vi "CRYGet Information for ActiveX.vi"() -> (2 "Limit Array Out":string, 3 "Sequence Array Out":string)   [LabVIEW 2013]
uses:
  CRYProject/CRYProject Editor Global.vi
panel:
  out "Array":string[](array[string])
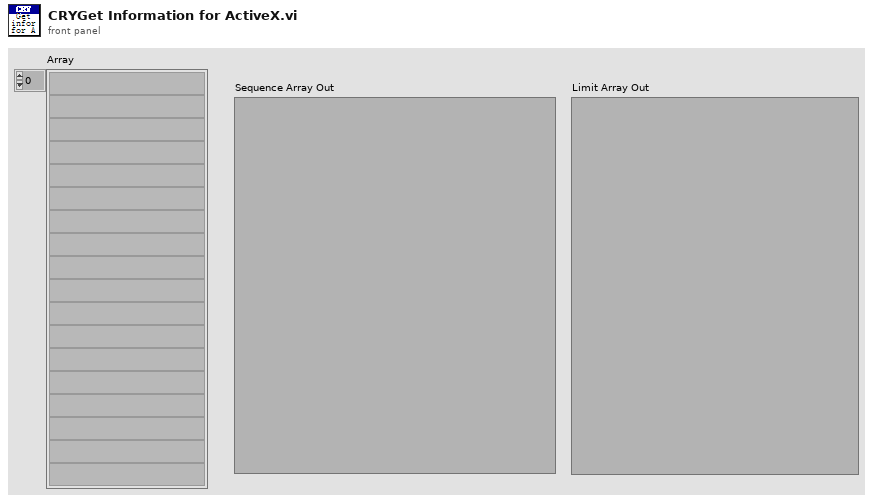
[diagram p1: front panel]
types:
  T1 = typedef "CRYStep.ctl" = cluster{"No.VI":i32, "Category":string, "StepName":string, "Seq setup flattened":string, "Comment":string, "Steps config.":bool[], "Jump config":i32[], "Start":dbl, "Increment":dbl, "Name":string, "Unit":string, "Y data":u16, "Y prefix":string, "Y dB ref":dbl, "Y unit":string, "Repeat State Array":cluster{"Start":dbl, "Increment":dbl, "Count":i32, "Num":i32}[]}
  T2 = typedef "CRYTS.ctl" = cluster{"No.TS":u16, "TS File Path":path, "TS Name":string, "EditStepName":string, "Steps":T1[], "New State":bool, "Change State":bool, "Flattened CurveLib Data":string, "Document Data":string, "EditStepNo":u16, "Operator Start File":string, "Sequence Type":string, "Sequence Language":string}
  T3 = typedef "CRYStimulus Cluster.ctl" = cluster{"StimulusType":string, "UseMLValArray":u16[], "ML_axisArray":u16[], "MLValLevelNameArray":string[], "Level(U)Array":dbl[], "Start(Stop)FreqArray":dbl[], "Start(Stop)AmpArray":dbl[], "StepResolutionArray":u16[], "Unit_Array":u16[], "DegValArray":dbl[], "DegUnitArray":string[], "Steps1":i32, "Cycle/step1(#)":u32, "Time/step1(s)":dbl, "Transition1":dbl, "SweepRate2":dbl, "Freq3(Hz)":dbl, "Steps3(#)":dbl, "Cycles3(#)":u32, "StepSize3":dbl, "wave time":string, "RMS_Value4":dbl, "Peak_Value4":dbl, "WavePath4":string, "RMS_unit4":string, "Peak_unit4":string, "wave Info":string, "dc_ctrl5_1":u16, "dc_ctrl5_2":u16, "dc_polar5":u16, "Max.Current":u16, "Steps5(#)":u32, "Time/Step5":dbl, "Level5":dbl, "StepsSize5Val":dbl, "StepSize5Unit":string, "SweepType":u16, "Fixed/Ratio6":u16, "Transition6":dbl, "Steps6(#)":dbl, "Cycle/Steps6(#)":u32, "Time/Steps6(s)":dbl, "Freq6(Hz)":dbl, "Difference6(Hz)":dbl, "Ratio6":string, "NoiseType7":u16, "Duration7(s)":dbl, "MinFreq7(Hz)":dbl, "MaxFreq7(Hz)":dbl, "MinFreq8(Hz)":dbl, "MaxFreq8(Hz)":dbl, "FreqRounding8":bool, "Duration8(s)":dbl, "Tones8":dbl, "RoundingVal8":dbl, "ApplyEQ":bool, "Duration(s)":dbl, "CustomStimulusName ":string, "Flatten Element Array":string[], "sine waves":cluster{"freq":dbl, "ampl":dbl, "cycles":dbl}[], "Channel Out":i32, "RatioVal6":dbl, "TabCtrl6":enum32{"Master Tone", "Slave Tone"}, "Signal Type Name":string, "Help":string, "Channel Sel":u16, "V on DUT":bool, "Output Imp":dbl, "Nominal Imp":dbl}
  T4 = typedef "CRYHardware Channel Info.ctl" = cluster{"ID":i32, "Name":string, "Digital":bool, "Input":bool, "Device Name":string, "Hardware Ch ID":u8, "Vmax (V)":dbl, "Latency (samples)":dbl, "Sampling Rate (Hz)":u32, "Bit Depth":u32, "Anti-aliasing Factor (%fs)":sgl, "DAQmx Channel":tag, "term config":i32, "Coupling":i32, "IEPE en":bool, "ASIOChannel Name":string, "Audio Driver":u16, "ASIOChannel Index":u8}
  T5 = typedef "CRYAcquisition Cluster.ctl" = cluster{"Mode":u16, "Name":string, "use ch name":bool, "Record Time":dbl, "hide rec":bool, "hide play":bool, "rec delay":dbl, "rec pad":dbl, "dcc units":i8, "sine gen setting":string, "scope_fft setting":string, "voltmeter setting":string, "rta setting":string, "trig offset(sec)":dbl, "triggered  record":bool, "trig level":dbl, "trig unit":u8, "trig slop":bool, "trig timeout(sec)":dbl, "add record":bool, "EQ":bool, "record table":string[][], "play table":string[][], "trig channel":string, "Help":string}
  T6 = typedef "CRYResult Cluster Array.ctl" = T7[]
  T7 = typedef "CRYResult Cluster.ctl" = cluster{"Name":string, "Margin":dbl, "unit":string, "Verdict":bool, "Limit":string, "Max/Min":string, "protected":bool, "Step No.":i32, "Test Info":string, "AutoProtect":bool}
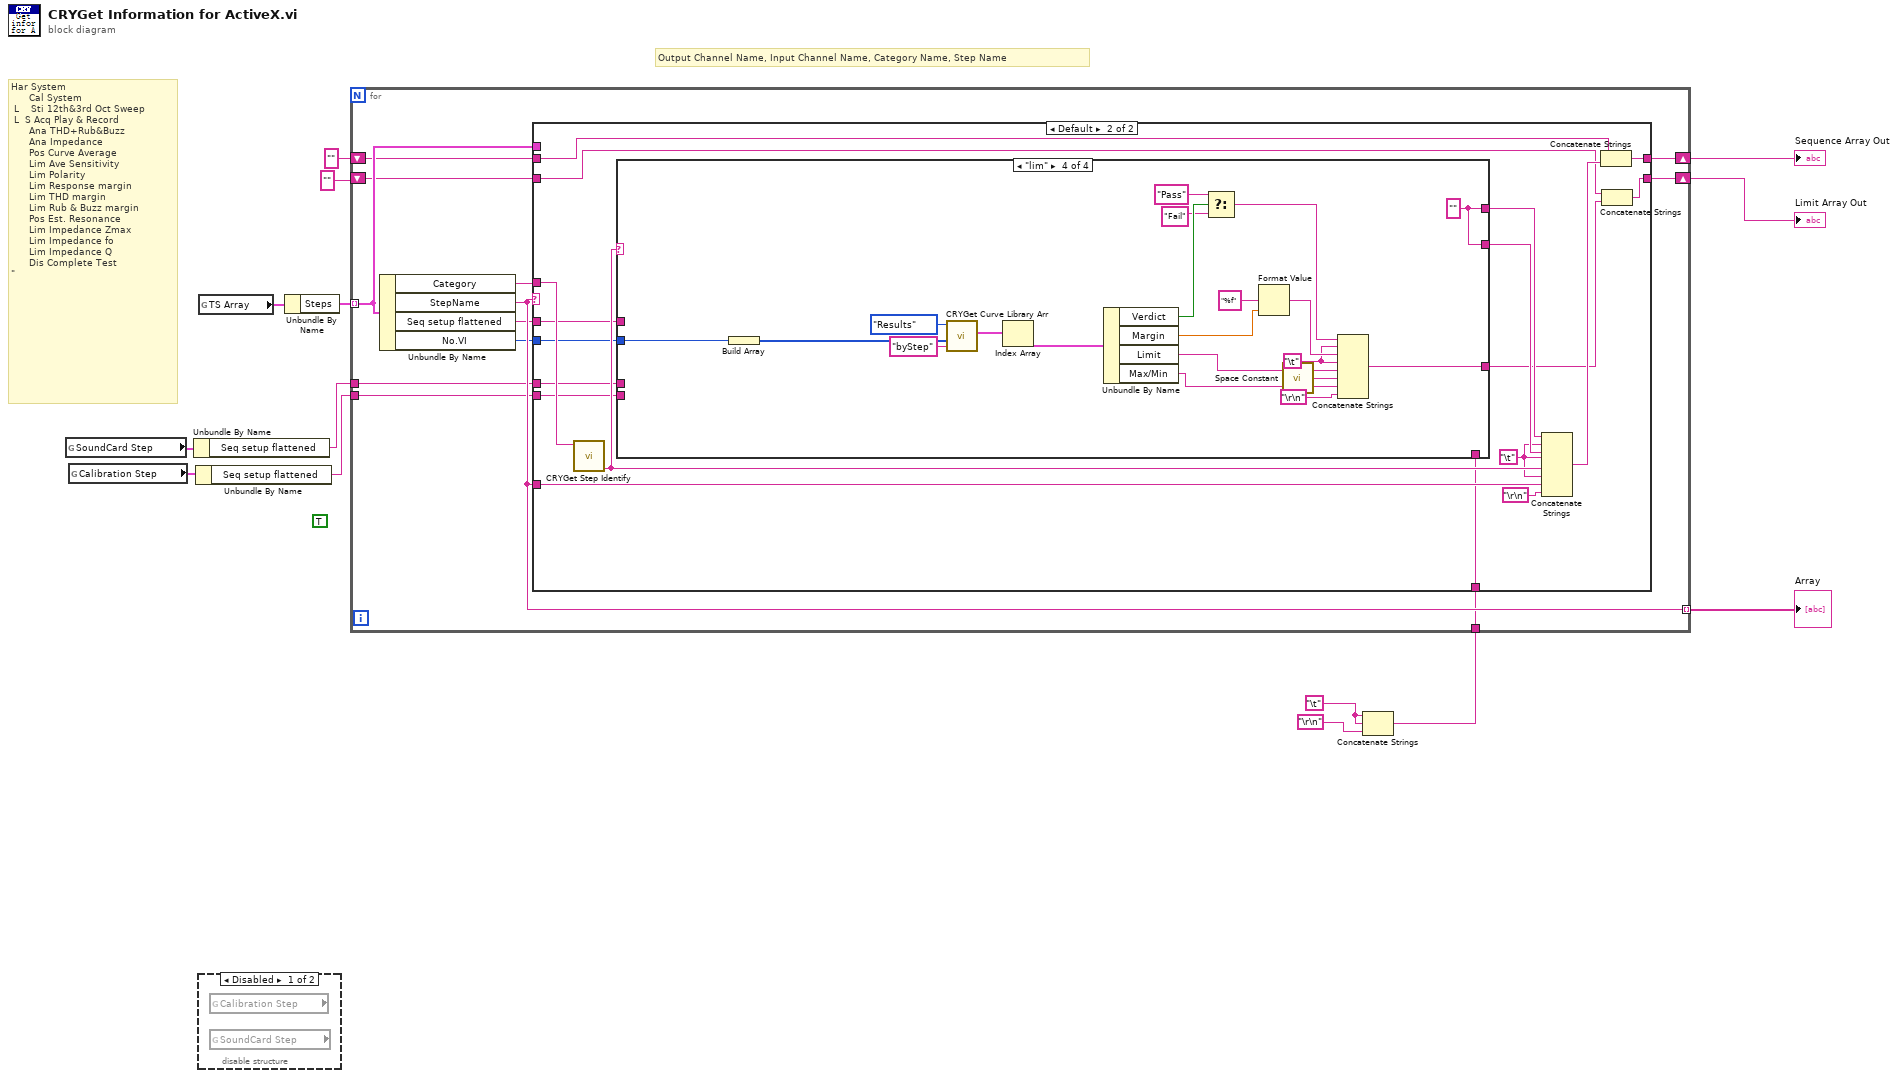
[diagram p0: block diagram]
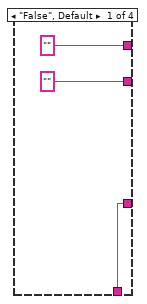
[diagram p4: hidden frame]
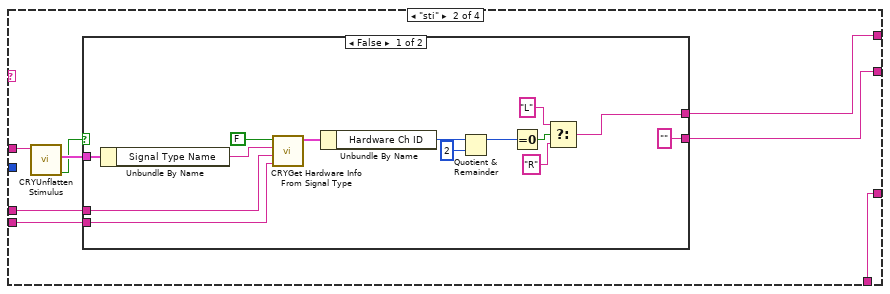
[diagram p5: hidden frame]
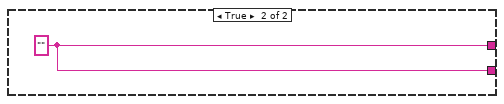
[diagram p6: hidden frame]
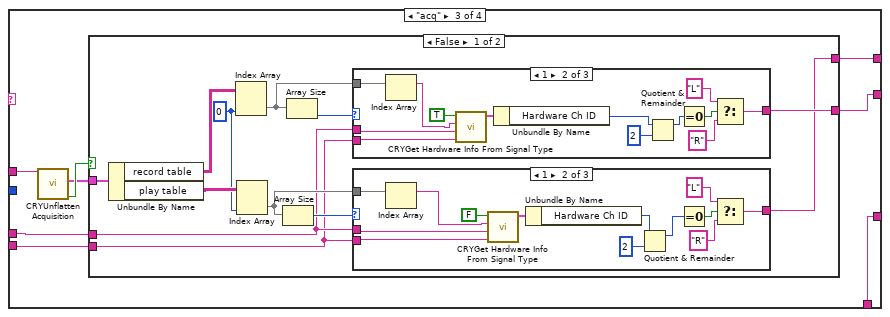
[diagram p7: hidden frame]
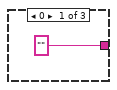
[diagram p8: hidden frame]
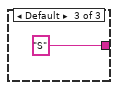
[diagram p9: hidden frame]
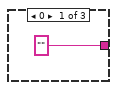
[diagram p10: hidden frame]
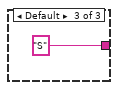
[diagram p11: hidden frame]
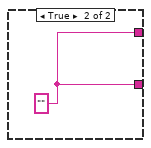
[diagram p12: hidden frame]
diagram:
  (unwired) TRUE ("Verdict")
  w1 = "\t"
  # "Output Channel Name, Input Channel Name, Category Name, Step Name"
  # "Har\tSystem\n  \t  \tCal\tSystem\n L\t  \tSti\t12th&3rd Oct Sweep\n L\t S\tAcq\tPlay & Record\n  \t  \tAna\tTHD+Rub&Buzz\n  \t  \tAna\tImpedance\n  \t  \tPos\tCurve Average\n  \t  \tLim\tAve Sensitivity\n  \t  \tLim\tPolarity\n  \t  \tLim\tResponse margin\n  \t  \tLim\tTHD margin\n  \t  \tLim\tRub & Buzz margin\n  \t  \tPos\tEst. Resonance\n  \t  \tLim\tImpedance Zmax\n  \t  \tLim\tImpedance fo\n  \t  \tLim\tImpedance Q\n  \t  \tDis\tComplete Test\n\""
  n1 = global read "CRYProject Editor Global.vi" "SoundCard Step"() -> (w9:T1)
  n2 = global read "CRYProject Editor Global.vi" "Calibration Step"() -> (w8:T1)
  n3 = Unbundle By Name(w9) -> ("Seq setup flattened"=w7:string)
  n4 = Unbundle By Name(w8) -> ("Seq setup flattened"=w6:string)
  n5 = global read "CRYProject Editor Global.vi" "TS Array"() -> (w14:T2)
  n6 = disable-structure shown="Disabled" {
    frame Disabled {
      n7 = global read "CRYProject Editor Global.vi" "Calibration Step"() -> ()  [unwired: 1 out]
      n8 = global read "CRYProject Editor Global.vi" "SoundCard Step"() -> ()  [unwired: 1 out]
    }
    frame Enabled {
    }
  }
  n9 = Unbundle By Name(w14) -> ("Steps"=w13:T1[])
  n10 = Concatenate Strings(w1, w1, "\r\n") -> (w3:string)
  n11 = for {
    tunnel: w13 -> [w26] mode=indexing
    shift-right: [w24] -> w11
    shift-left: "" ("Identfier") -> [w25]
    tunnel: [w23] -> w10 mode=indexing
    tunnel: w7 -> [w20]
    tunnel: w6 -> [w19]
    shift-right: [w17] -> w4
    shift-left: "" ("Identfier") -> [w16]
    tunnel: w3 -> [w15]
    n12 = Unbundle By Name(w26) -> ("Category"=w22:string, "StepName"=w23:string, "Seq setup flattened"=w21:string, "No.VI"=w18:i32)
    n13 = case shown="Default" w23 {
      tunnel: w26 -> [_ _]
      tunnel: w25 -> [w28 w39]
      tunnel: [w28 w38] -> w24
      tunnel: w23 -> [_ w42]
      tunnel: w22 -> [_ w37]
      tunnel: w21 -> [_ w36]
      tunnel: w20 -> [_ w35]
      tunnel: w19 -> [_ w34]
      tunnel: w18 -> [_ w33]
      tunnel: [w27 w31] -> w17
      tunnel: w16 -> [w27 w30]
      tunnel: w15 -> [_ w29]
      frame "End", "Start" {
      }
      frame Default {
        w43 = "\t"
        n14 = call "CRYGet Step Identify.vi"("Category Name In"=w37) -> ("Identfier"=w44:string)  [unwired: 3 in, 7 out]
        n15 = case shown="\"lim\"" w44 {
          tunnel: ["" ("Identfier") w54 w75 w143] -> w46
          tunnel: ["" ("Identfier") w53 w74 w143] -> w45
          tunnel: w36 -> [_ w57 w77 _]
          tunnel: w35 -> [_ w52 w79 _]
          tunnel: w34 -> [_ w51 w78 _]
          tunnel: w33 -> [_ _ _ w141]
          tunnel: [w47 w50 w73 w128] -> w32
          tunnel: w29 -> [w47 w50 w73 _]
          frame "False", Default {
          }
          frame "sti" {
            n16 = call "CRYUnflatten Stimulus.vi"("Flatten Stimulus"=w57) -> ("Error?"=w55:bool, "Stimulus"=w56:T3)  [unwired: 8 in, 1 out]
            n17 = case shown="False" w55 {
              tunnel: w56 -> [w71 _]
              tunnel: [w63 w72] -> w54
              tunnel: ["" ("Identfier") w72] -> w53
              tunnel: w52 -> [w62 _]
              tunnel: w51 -> [w61 _]
              frame False {
                n18 = Unbundle By Name(w71) -> ("Signal Type Name"=w69:string)
                n19 = call "CRYGet Hardware Info From Signal Type.vi"("Calibration In"=w61, "Hardware In"=w62, "Signal Type"=w69, "In/Out?"=FALSE) -> ("Channel Info Out"=w67:T4)  [unwired: 5 in, 2 out]
                n20 = Unbundle By Name(w67) -> ("Hardware Ch ID"=w60:u8)
                n21 = Quotient & Remainder(x=w60, y=u8 2) -> (x-y*floor(x/y)=w58:u8)  [unwired: 1 out]
                n22 = Equal To 0?(x=w58) -> (x = 0?=w66:bool)
                n23 = Select(t="L" ("Identfier"), s=w66, f="R" ("Identfier")) -> (s? t:f=w63:string)
              }
              frame True {
                w72 = "" ("Identfier")
              }
            }
          }
          frame "acq" {
            n24 = call "CRYUnflatten Acquisition.vi"("Flatten Acquisition"=w77) -> ("Error?"=w80:bool, "Acquisition"=w76:T5)  [unwired: 8 in, 1 out]
            n25 = case shown="False" w80 {
              tunnel: w76 -> [w92 _]
              tunnel: [w91 w123] -> w74
              tunnel: [w81 w123] -> w75
              tunnel: w79 -> [w83 _]
              tunnel: w78 -> [w82 _]
              frame False {
                w88 = 0 ("disabled index (col)")
                n26 = Unbundle By Name(w92) -> ("record table"=w90:string[][], "play table"=w89:string[][])
                n27 = Index Array(array=w90, index (col)=w88) -> (element=w87:string[])  [unwired: 1 in]
                n28 = Index Array(array=w89, index (col)=w88) -> (element=w84:string[])  [unwired: 1 in]
                n29 = Array Size(array=w84) -> (size(s)=w85:i32)
                n30 = Array Size(array=w87) -> (size(s)=w86:i32)
                n31 = case shown="1" w86 {
                  tunnel: ["" ("Identfier") w116 "S" ("Identfier")] -> w91
                  tunnel: w83 -> [_ w115 _]
                  tunnel: w82 -> [_ w114 _]
                  tunnel: w87 -> [_ w113 _]
                  frame 0 {
                  }
                  frame 1 {
                    n32 = Index Array(array=w113) -> (element=w112:string)  [unwired: 1 in]
                    n33 = call "CRYGet Hardware Info From Signal Type.vi"("Calibration In"=w114, "Hardware In"=w115, "Signal Type"=w112, "In/Out?"=TRUE) -> ("Channel Info Out"=w120:T4)  [unwired: 5 in, 2 out]
                    n34 = Unbundle By Name(w120) -> ("Hardware Ch ID"=w110:u8)
                    n35 = Quotient & Remainder(x=w110, y=u8 2) -> (x-y*floor(x/y)=w109:u8)  [unwired: 1 out]
                    n36 = Equal To 0?(x=w109) -> (x = 0?=w119:bool)
                    n37 = Select(t="L" ("Identfier"), s=w119, f="R" ("Identfier")) -> (s? t:f=w116:string)
                  }
                  frame Default {
                  }
                }
                n38 = case shown="1" w85 {
                  tunnel: ["" ("Identfier") w101 "S" ("Identfier")] -> w81
                  tunnel: w83 -> [_ w100 _]
                  tunnel: w82 -> [_ w99 _]
                  tunnel: w84 -> [_ w98 _]
                  frame 0 {
                  }
                  frame 1 {
                    n39 = Index Array(array=w98) -> (element=w97:string)  [unwired: 1 in]
                    n40 = call "CRYGet Hardware Info From Signal Type.vi"("Calibration In"=w99, "Hardware In"=w100, "Signal Type"=w97, "In/Out?"=FALSE) -> ("Channel Info Out"=w105:T4)  [unwired: 5 in, 2 out]
                    n41 = Unbundle By Name(w105) -> ("Hardware Ch ID"=w95:u8)
                    n42 = Quotient & Remainder(x=w95, y=u8 2) -> (x-y*floor(x/y)=w94:u8)  [unwired: 1 out]
                    n43 = Equal To 0?(x=w94) -> (x = 0?=w104:bool)
                    n44 = Select(t="L" ("Identfier"), s=w104, f="R" ("Identfier")) -> (s? t:f=w101:string)
                  }
                  frame Default {
                  }
                }
              }
              frame True {
                w123 = "" ("Identfier")
              }
            }
          }
          frame "lim" {
            w127 = "\t"
            w143 = "" ("Identfier")
            n45 = Build Array(w141) -> (w140:i32[])
            n46 = call "CRYGet Curve Library Arr.vi"("Index"=w140, "sOption"="byStep", "Type In"=enum16{"Curves", "Values", "Results", "WFM"}."Results") -> ("Results"=w138:T6)  [unwired: 6 in, 2 out]
            n47 = Index Array(array=w138) -> (element=w137:T7)  [unwired: 1 in]
            n48 = Unbundle By Name(w137) -> ("Verdict"=w136:bool, "Margin"=w131:dbl, "Limit"=w129:string, "Max/Min"=w125:string)
            n49 = Select(t="Pass" ("Identfier"), s=w136, f="Fail" ("Identfier")) -> (s? t:f=w133:string)
            n50 = Format Value(format string="%f", value (0)=w131) -> (output string=w130:string)  [unwired: 1 in]
            n51 = call <vilib>:"Space Constant.vi"() -> ("String"=w124:string)
            n52 = Concatenate Strings(w133, w127, w130, w127, w129, w124, w125, "\r\n") -> (w128:string)
          }
        }
        n53 = Concatenate Strings(w46, w43, w45, w43, w44, w43, w42, "\r\n") -> (w40:string)
        n54 = Concatenate Strings(w39, w40) -> (w38:string)
        n55 = Concatenate Strings(w30, w32) -> (w31:string)
      }
    }
  }
  "Sequence Array Out" <- w11
  "Array" <- w10
  "Limit Array Out" <- w4
